vi "Read Input Data Word.vi"(8 "error in (no error)":errorcluster {"code" format="%.0x"}, 9 "ValBufferSize":i32=2048, 10 "ChannelList":string, 11 "instrument handle":refnum<k15>) -> (0 "error out":errorcluster {"code" format="%.0x"}, 1 "ValActualSize":i32, 2 "Val":i32[](array[numeric]), 3 "instrument handle out":refnum<k15>)   [LabVIEW 2020, in "Keysight DAQ970.lvlib"]
doc: "Configures channel for input and immediately gets the 16-bit word data of the specified digital channels (s01 only). Does not redefine the scan list."
uses:
  Keysight DAQ970.lvlib
  KtDAQ970.dll
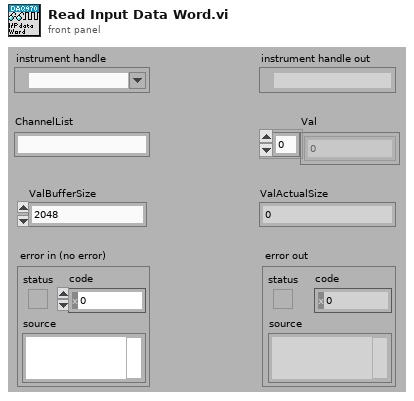
[diagram p1: front panel]
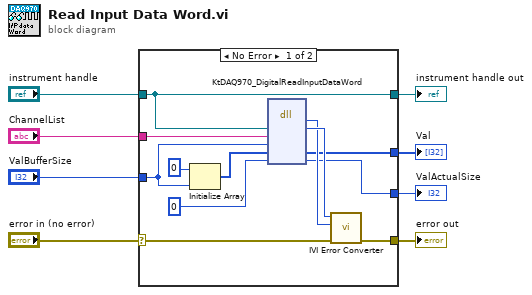
[diagram p0: block diagram]
diagram:
  n1 = case shown="No Error" "error in (no error)" {
    selector: "error in (no error)" -> [w18 w22]
    tunnel: [w17 w22] -> w8
    tunnel: "instrument handle" -> [w10 w21]
    tunnel: "ChannelList" -> [w16 _]
    tunnel: "ValBufferSize" -> [w9 _]
    tunnel: [w13 _] -> w3
    tunnel: [w11 _] -> w2
    tunnel: [w10 w21] -> w1
    frame No Error {
      n2 = Initialize Array(0 ("element"), w9) -> (w15:i32[])
      n3 = dll-call lib="KtDAQ970**.dll" fn="KtDAQ970_DigitalReadInputDataWord"("Vi"=w10, "ChannelList"=w16, "ValBufferSize"=w9, "Val"=w15, "ValActualSize"=0) -> (w19:i32, "Vi"=w20:u32, "Val"=w13:i32[], "ValActualSize"=w11:i32)  [unwired: 5 in, 2 out]
      n4 = call "IVI Error Converter.vi"("error in (no error)"=w18, "IVI error code (0)"=w19, "instrument handle"=w20) -> ("error out"=w17:errorcluster)  [unwired: 7 in, 1 out]
    }
    frame Error {
    }
  }
  "error out" <- w8
  "instrument handle out" <- w1
  "Val" <- w3
  "ValActualSize" <- w2
